vi "Global Para.vi"() -> ()   [LabVIEW 2014]
panel:
  out "Goal":bool
  in  "Log Data":dbl[][](array[numeric])
  out "Init Time":timestamp
  in  "Terget Position":dbl
  out "SET?":bool
  out "Current Position （mm  /  °）":dbl
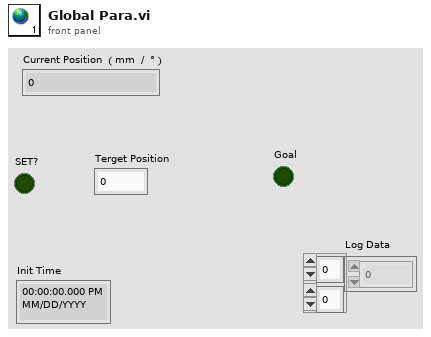
[diagram p1: front panel]
diagram:
